vi "Swop_Instrument_Positions.vi"() -> (0 "error out":errorcluster, 4 "Path":path)   [LabVIEW 2015]
panel:
  out "File Changed":bool
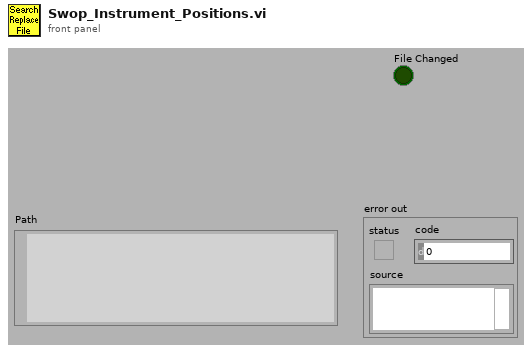
[diagram p1: front panel]
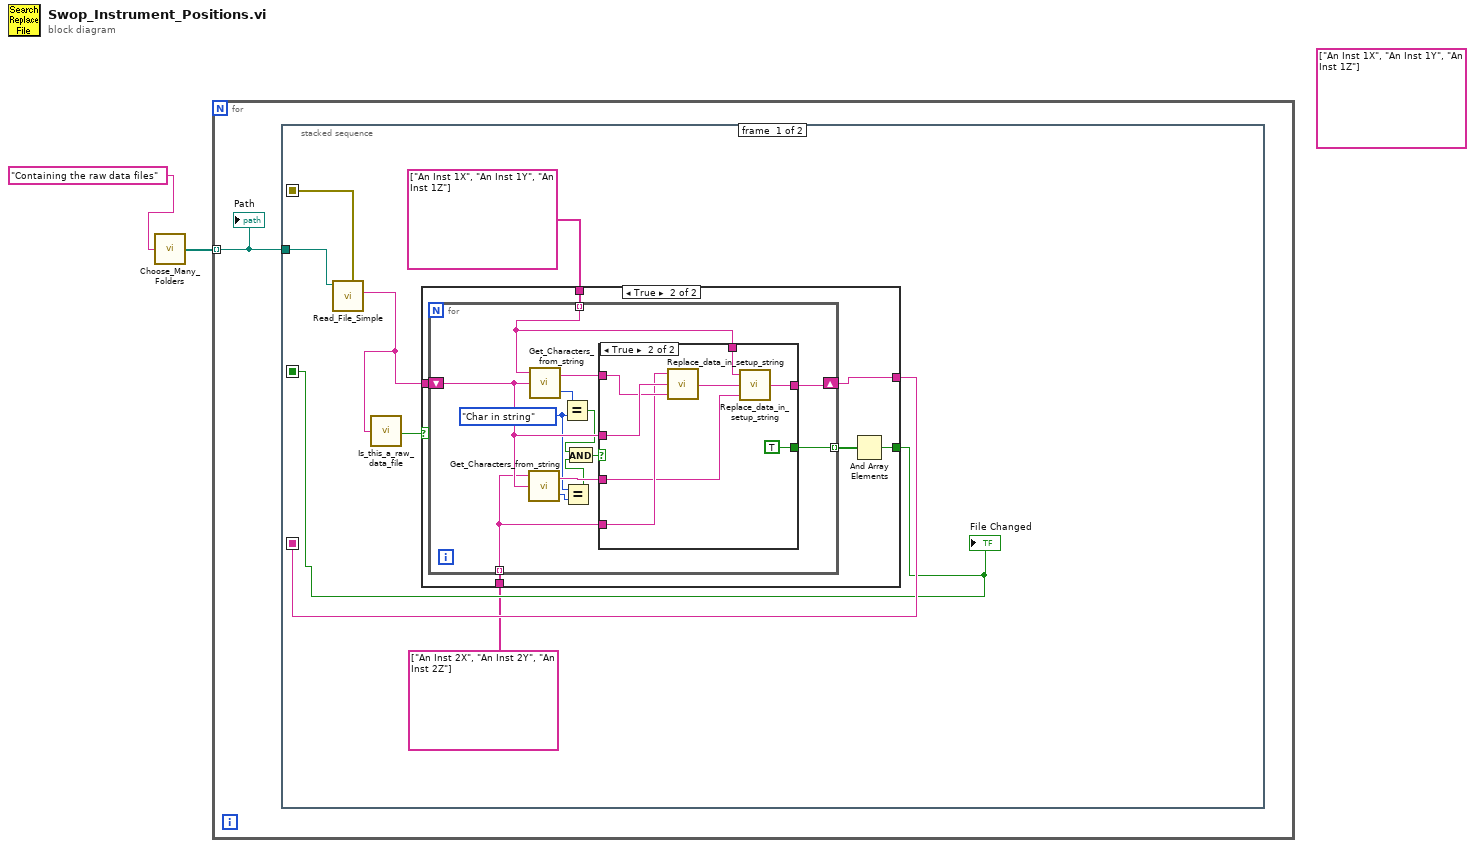
[diagram p0: block diagram]
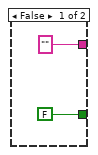
[diagram p2: hidden frame]
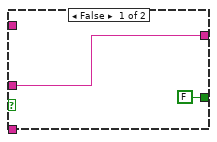
[diagram p3: hidden frame]
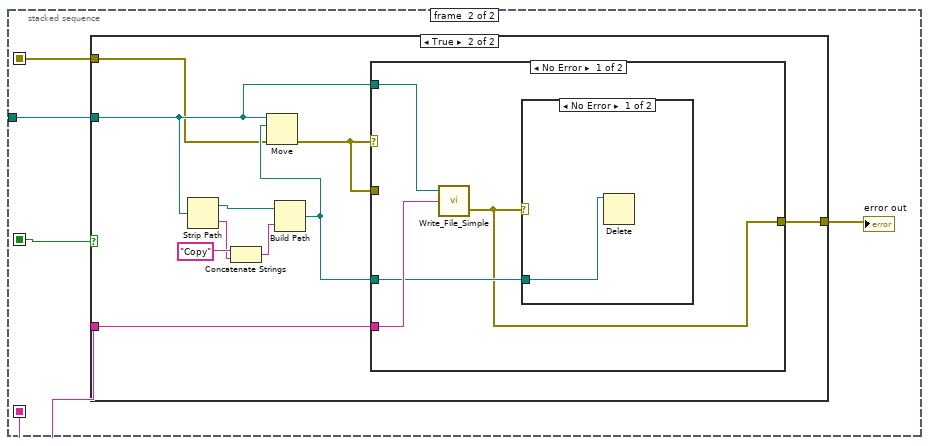
[diagram p4: hidden frame]
diagram:
  (unwired) string[] ["An Inst 1X", "An Inst 1Y", "An Inst 1Z"]
  n1 = call "Choose_Many_Folders.vi"("Purpose of choosing folder"="Containing the raw data files") -> ("Files"=w1:path[])
  n2 = for {
    tunnel: w1 -> [w3] mode=indexing
    n3 = stacked-sequence {
      seq-local: [w10 _] -> [_ w43]
      seq-local: [w8 _] -> [_ w45]
      seq-local: [w7 _] -> [_ w44]
      tunnel: w3 -> [w11 w47]
      frame #0 {
        n4 = call "Read_File_Simple.vi"("Filename"=w11) -> ("error out"=w10:errorcluster, "string"=w6:string)  [unwired: 4 in, 4 out]
        n5 = call "Is_this_a_raw_data_file.vi"("character string"=w6) -> ("Raw Dat File?"=w5:bool)  [unwired: 2 out]
        n6 = case shown="True" w5 {
          tunnel: string[] ["An Inst 1X", "An Inst 1Y", "An Inst 1Z"] -> [_ w19]
          tunnel: ["" ("string") w18] -> w8
          tunnel: [FALSE w16] -> w7
          tunnel: w6 -> [_ w15]
          tunnel: string[] ["An Inst 2X", "An Inst 2Y", "An Inst 2Z"] -> [_ w14]
          frame False {
          }
          frame True {
            n7 = for {
              shift-right: [w32] -> w18
              shift-left: w15 -> [w29]
              tunnel: w19 -> [w27] mode=indexing
              tunnel: [w30] -> w17 mode=indexing
              tunnel: w14 -> [w28] mode=indexing
              w23 = enum16{"Char in string", "Char not in string"}."Char in string" ("Status")
              n8 = call "Get_Characters_from_string.vi"("Input string"=w29, "Variable name"=w28) -> ("Status"=w24:enum16{"Char in string", "Char not in string"}, "Value"=w26:string)  [unwired: 1 in]
              n9 = call "Get_Characters_from_string.vi"("Input string"=w29, "Variable name"=w27) -> ("Status"=w25:enum16{"Char in string", "Char not in string"}, "Value"=w31:string)  [unwired: 1 in]
              n10 = Equal?(x=w25, y=w23) -> (x = y?=w21:bool)
              n11 = Equal?(x=w23, y=w24) -> (x = y?=w22:bool)
              n12 = And(x=w21, y=w22) -> (x .and. y?=w20:bool)
              n13 = case shown="True" w20 {
                tunnel: w27 -> [_ w42]
                tunnel: w29 -> [w34 w41]
                tunnel: [w34 w40] -> w32
                tunnel: w31 -> [_ w38]
                tunnel: [FALSE TRUE] -> w30
                tunnel: w28 -> [_ w36]
                tunnel: w26 -> [_ w35]
                frame False {
                }
                frame True {
                  n14 = call "Replace_data_in_setup_string.vi"("New data string"=w38, "Input string"=w41, "Variable name"=w36) -> ("Appended string"=w39:string)
                  n15 = call "Replace_data_in_setup_string.vi"("New data string"=w35, "Input string"=w39, "Variable name"=w42) -> ("Appended string"=w40:string)
                }
              }
            }
            n16 = And Array Elements(Boolean array=w17) -> (logical AND=w16:bool)
          }
        }
        "File Changed" <- w7
      }
      frame #1 {
        n17 = case shown="True" w44 {
          tunnel: w47 -> [_ w54]
          tunnel: w45 -> [_ w53]
          tunnel: [w48 w51] -> w46
          tunnel: w43 -> [w48 w49]
          frame False {
          }
          frame True {
            n18 = Strip Path(path=w54) -> (stripped path=w55:path, name=w57:string)
            n19 = Concatenate Strings("Copy" ("name or relative path"), w57) -> (w56:string)
            n20 = Build Path(base path=w55, name or relative path=w56) -> (appended path=w52:path)
            n21 = Move(source path=w54, error in=w49, 10:w52) -> (error out=w50:errorcluster)  [unwired: 2 in, 2 out]
            n22 = case shown="No Error" w50 {
              tunnel: w54 -> [w62 _]
              tunnel: w53 -> [w61 _]
              tunnel: w52 -> [w60 _]
              tunnel: [w59 w64] -> w51
              tunnel: w50 -> [_ w64]
              frame No Error {
                n23 = call "Write_File_Simple.vi"("character string"=w61, "file path"=w62) -> ("error out"=w59:errorcluster)  [unwired: 1 in, 1 out]
                n24 = case shown="No Error" w59 {
                  tunnel: w60 -> [w63 _]
                  frame No Error {
                    n25 = Delete(path (use dialog)=w63) -> ()  [unwired: 4 in, 3 out]
                  }
                  frame Error {
                  }
                }
              }
              frame Error {
              }
            }
          }
        }
        "error out" <- w46
      }
    }
    "Path" <- w3
  }
